vi "Iteration.vi"(7 "Variables in":refnum<class "Variables.lvclass">, 8 "error in (no error)":errorcluster, 9 "Transition":bool, 11 "State in":refnum<class "State.lvclass">) -> (0 "error out":errorcluster, 1 "Iteration Result":T1, 3 "State out":refnum<class "State.lvclass">, 5 "Variables":refnum<class "Variables.lvclass">)   [LabVIEW 2020, in "VolatusSeq.lvlib" / "State.lvclass"]
uses:
  State.lvclass
  State.lvclass/State.ctl
  Variables/Variables.lvclass
  Iteration Result.ctl
  VolatusSeq.lvlib
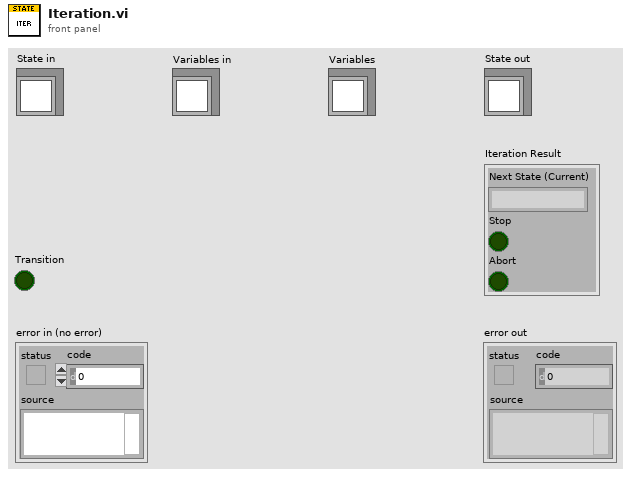
[diagram p1: front panel]
types:
  T1 = typedef "VolatusSeq.lvlib/Iteration Result.ctl" = cluster{"Next State (Current)":string, "Stop":bool, "Abort":bool}
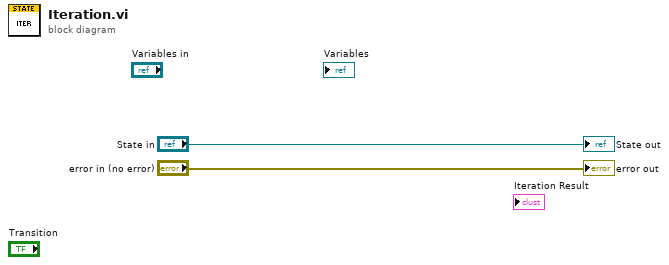
[diagram p0: block diagram]
diagram:
  "error out" <- "error in (no error)"
  "State out" <- "State in"
